vi "DisplayMessageAsync.vi"(8 "error in (no error)":errorcluster, 11 "Message":string) -> ()   [LabVIEW 2013]
doc: "Asynchronously call DisplayMessage.vi with the given input. The caller process will not be blocked."
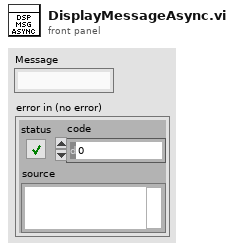
[diagram p1: front panel]
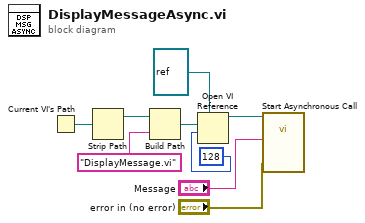
[diagram p0: block diagram]
diagram:
  n1 = Current VI's Path() -> (path=w7:path)
  n2 = Strip Path(path=w7) -> (stripped path=w8:path)  [unwired: 1 out]
  n3 = Build Path(base path=w8, name or relative path="DisplayMessage.vi") -> (appended path=w6:path)
  n4 = Open VI Reference(type specifier VI Refnum (for type only)=refnum<vi> refnum, vi path=w6, options=128) -> (vi reference=w4:refnum<vi>)  [unwired: 3 in, 1 out]
  n5 = call-by-ref "Start Asynchronous Call"(reference=w4, "error in (no error)"="error in (no error)", "Message"="Message") -> ()  [unwired: 11 in, 2 out]
